vi "Plot_FFT_Env.vi"(0 "FFT input":T1, 1 "x > sample read?":bool, 2 "last order plot":sgl, 5 "rotation speed":sgl, 7 "samples to plot":i32, 9 "Array in":dbl[][](array[numeric]), 11 "error in (no error)":errorcluster, 12 "Array":dbl[](array[numeric]), 13 "Numeric":i32) -> (4 "3D Plot lvclass Array out":refnum<class "3D Plot Datatype.lvclass">[](array[class]), 6 "Array out":dbl[][](array[numeric]), 15 "error out":errorcluster)   [LabVIEW 2025]
uses:
  <vilib>/Math Plots/3D Math Plots/3D Contour/3D Contour Datatype/3D Contour Datatype.lvclass
  <vilib>/Math Plots/3D Math Plots/3D Contour/3D Contour Datatype/Public/Plot Helper (Vector).vi
  <vilib>/Math Plots/3D Math Plots/3D Plot/3D Plot Datatype/3D Plot Datatype.lvclass
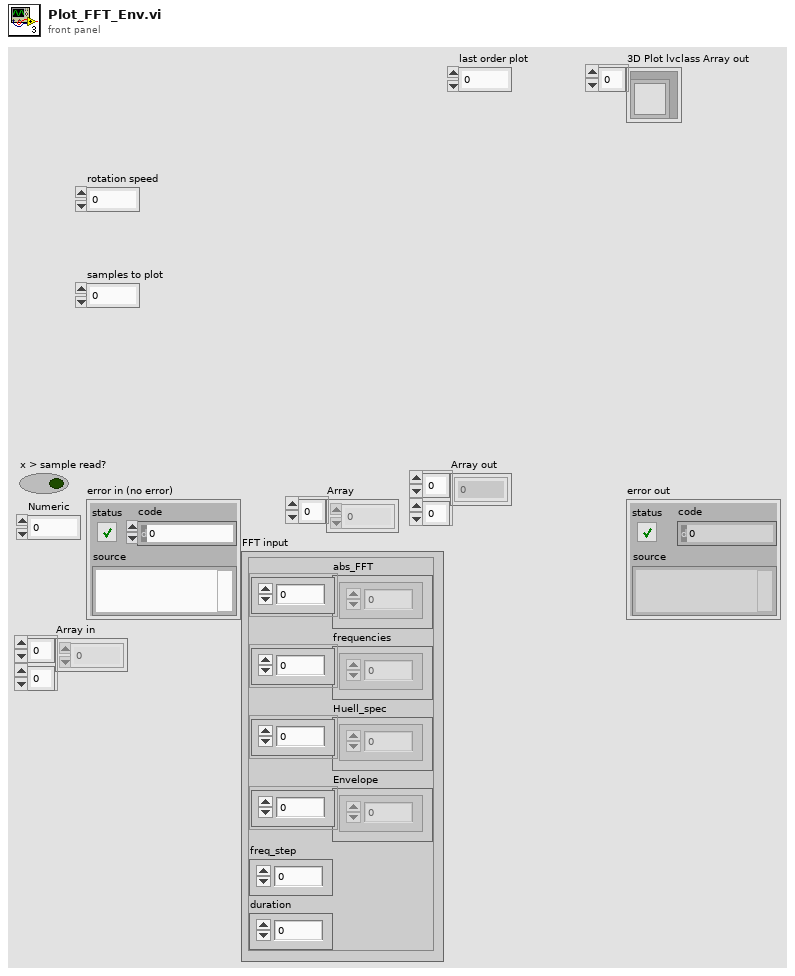
[diagram p1: front panel]
types:
  T1 = cluster{"abs_FFT":dbl[], "frequencies":dbl[], "Huell_spec":dbl[], "Envelope":dbl[], "freq_step":dbl, "duration":dbl}
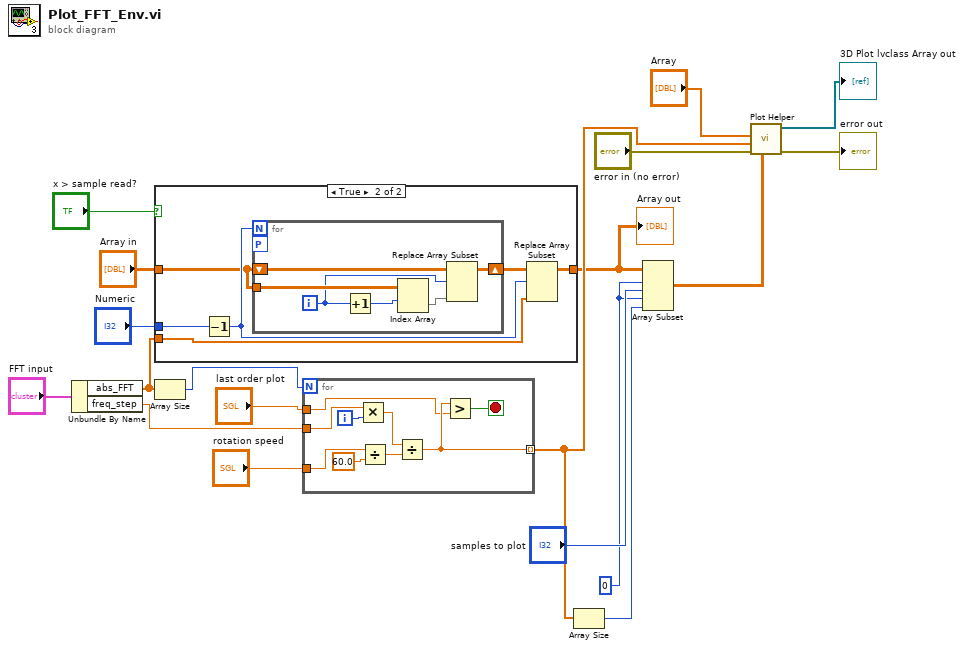
[diagram p0: block diagram]
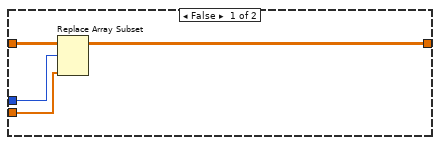
[diagram p2: hidden frame]
diagram:
  w6 = 0 ("length")
  n1 = Unbundle By Name("FFT input") -> ("abs_FFT"=w2:dbl[], "freq_step"=w7:dbl)
  n2 = case shown="True" "x > sample read?" {
    tunnel: "Array in" -> [w23 w24]
    tunnel: w2 -> [w21 w28]
    tunnel: "Numeric" -> [w22 w27]
    tunnel: [w20 w25] -> w4
    frame False {
      n3 = Replace Array Subset(array=w23, new element=w21, index (row)=w22) -> (w20:dbl[][])  [unwired: 1 in]
    }
    frame True {
      n4 = Decrement(x=w27) -> (x-1=w26:i32)
      n5 = for {
        N: w26 -> [_]
        tunnel: w24 -> [w35]
        shift-right: [w30] -> w29
        shift-left: w24 -> [w32]
        workers-P: _ -> [_]
        i -> [w31]
        n6 = Increment(x=w31) -> (x+1=w34:i32)
        n7 = Index Array(array=w35, index (row)=w34) -> (element=w33:dbl[])  [unwired: 1 in]
        n8 = Replace Array Subset(array=w32, new element=w33, index (row)=w31) -> (w30:dbl[][])  [unwired: 1 in]
      }
      n9 = Replace Array Subset(array=w29, new element=w28, index (row)=w26) -> (w25:dbl[][])  [unwired: 1 in]
    }
  }
  "Array out" <- w4
  n10 = Array Size(array=w2) -> (size(s)=w12:i32)
  n11 = for {
    N: w12 -> [_]
    tunnel: w7 -> [w36]
    tunnel: [w39] -> w13 mode=indexing
    tunnel: "rotation speed" -> [w40]
    tunnel: "last order plot" -> [w38]
    i -> [w44]
    stop <- w37 stop-if-true
    n12 = Multiply(x=w36, y=w44) -> (x*y=w41:dbl)
    n13 = Divide(x=w40, y=sgl 60.0) -> (x/y=w42:sgl)
    n14 = Divide(x=w41, y=w42) -> (x/y=w39:dbl)
    n15 = Greater?(x=w39, y=w38) -> (0:w37:bool)
  }
  n16 = Array Size(array=w13) -> (size(s)=w14:i32)
  n17 = Array Subset(array=w4, index (row)=w6, length (row)="samples to plot", index (col)=w6, length (col)=w14) -> (w15:dbl[][])
  n18 = call-poly <vilib>:"Plot Helper.vi"("z matrix"=w15, "error in (no error)"="error in (no error)", "y vector"=w13, "x vector"="Array") -> ("error out"=→"error out":errorcluster, "3D Plot lvclass Array out"=→"3D Plot lvclass Array out":refnum<class "3D Plot Datatype.lvclass">[])  [unwired: 2 in, 4 out]
